vi "Gyro Drive Straight.vi"   [LabVIEW 2015]
uses:
  <vilib>/addons/control/pid/pid.llb/PID (DBL).vi
  <vilib>/addons/control/pid/NI_PID_pid.lvlib
types:
  T1 = cluster{"proportional gain (Kc)":dbl, "integral time (Ti, min)":dbl, "derivative time (Td, min)":dbl}
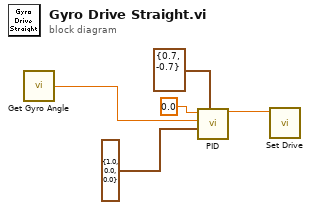
[diagram p0: block diagram]
diagram:
  n1 = call "Get Gyro Angle.vi"() -> ("Angle"=w5:dbl)  [unwired: 3 in]
  n2 = call-poly <vilib>:"PID.vi"("output range"=cluster{"output high":dbl, "output low":dbl} {"output high"=0.7, "output low"=-0.7}, "PID gains"=T1 {"proportional gain (Kc)"=1.0, "integral time (Ti, min)"=0.0, "derivative time (Td, min)"=0.0}, "process variable"=w5, "setpoint"=0.0) -> ("output"=w3:dbl)  [unwired: 6 in, 1 out]
  n3 = call "Set Drive.vi"("X axis value"=w3) -> ()  [unwired: 11 in]
